vi "axis to can.vi"(4 "wej  ID":T4, 7 "output cluster 3":T1 {"zadany" format="%<%H:%M:%S\n%x>T"}, 10 "wej wagi":T3, 11 "wej ster":cluster{"Y axis":i32, "X axis":i32}) -> (0 "array of cans":T5[](array[typedef]) {"type" items=["CAN Data", "CAN Remote"]; "identifier" format="%.0x"}, 1 "current time":timestamp format="%<%I:%M:%S %p\n%x>T", 2 "pierwsz ramka":T5 {"type" items=["CAN Data", "CAN Remote"]; "identifier" format="%.0x"}, 3 "druga ramka":T5 {"type" items=["CAN Data", "CAN Remote"]; "identifier" format="%.0x"}, 5 "wyj pred":cluster{u16, u16, u16, u16, u16, u16} {"?" scale=0.0..65000.0; "?" scale=0.0..65000.0; "?" scale=0.0..65000.0; "?" scale=0.0..65000.0; "?" scale=0.0..65000.0; "?" scale=0.0..65000.0}, 6 "output cluster 2":T2, 9 "wyœlij":bool=TRUE)   [LabVIEW 2014]
uses:
  CANFrameControl.ctl
panel:
  in  "reset":bool
  out "x-y":dbl
  out "Time has Elapsed":bool
  out "Elapsed Time (s)":dbl
  out "zadany czas":bool
  out "AUTO ?":bool
  out "P 10":dbl(slide) scale=-66000.0..66000.0
  out "L 10":dbl(slide) scale=-66000.0..66000.0
  out "L 9":dbl(slide) scale=-66000.0..66000.0
  out "L 8":dbl(slide) scale=-66000.0..66000.0
  out "P 9":dbl(slide) scale=-66000.0..66000.0
  out "P 8":dbl(slide) scale=-66000.0..66000.0
  out "P 7":dbl(slide) scale=-66000.0..66000.0
  out "P 6":dbl(slide) scale=-66000.0..66000.0
  out "L 7":dbl(slide) scale=-66000.0..66000.0
  out "L 6":dbl(slide) scale=-66000.0..66000.0
  out "P 5":dbl(slide) scale=-66000.0..66000.0
  out "L 5":dbl(slide) scale=-66000.0..66000.0
  out "P 4":dbl
  out "L 4":dbl
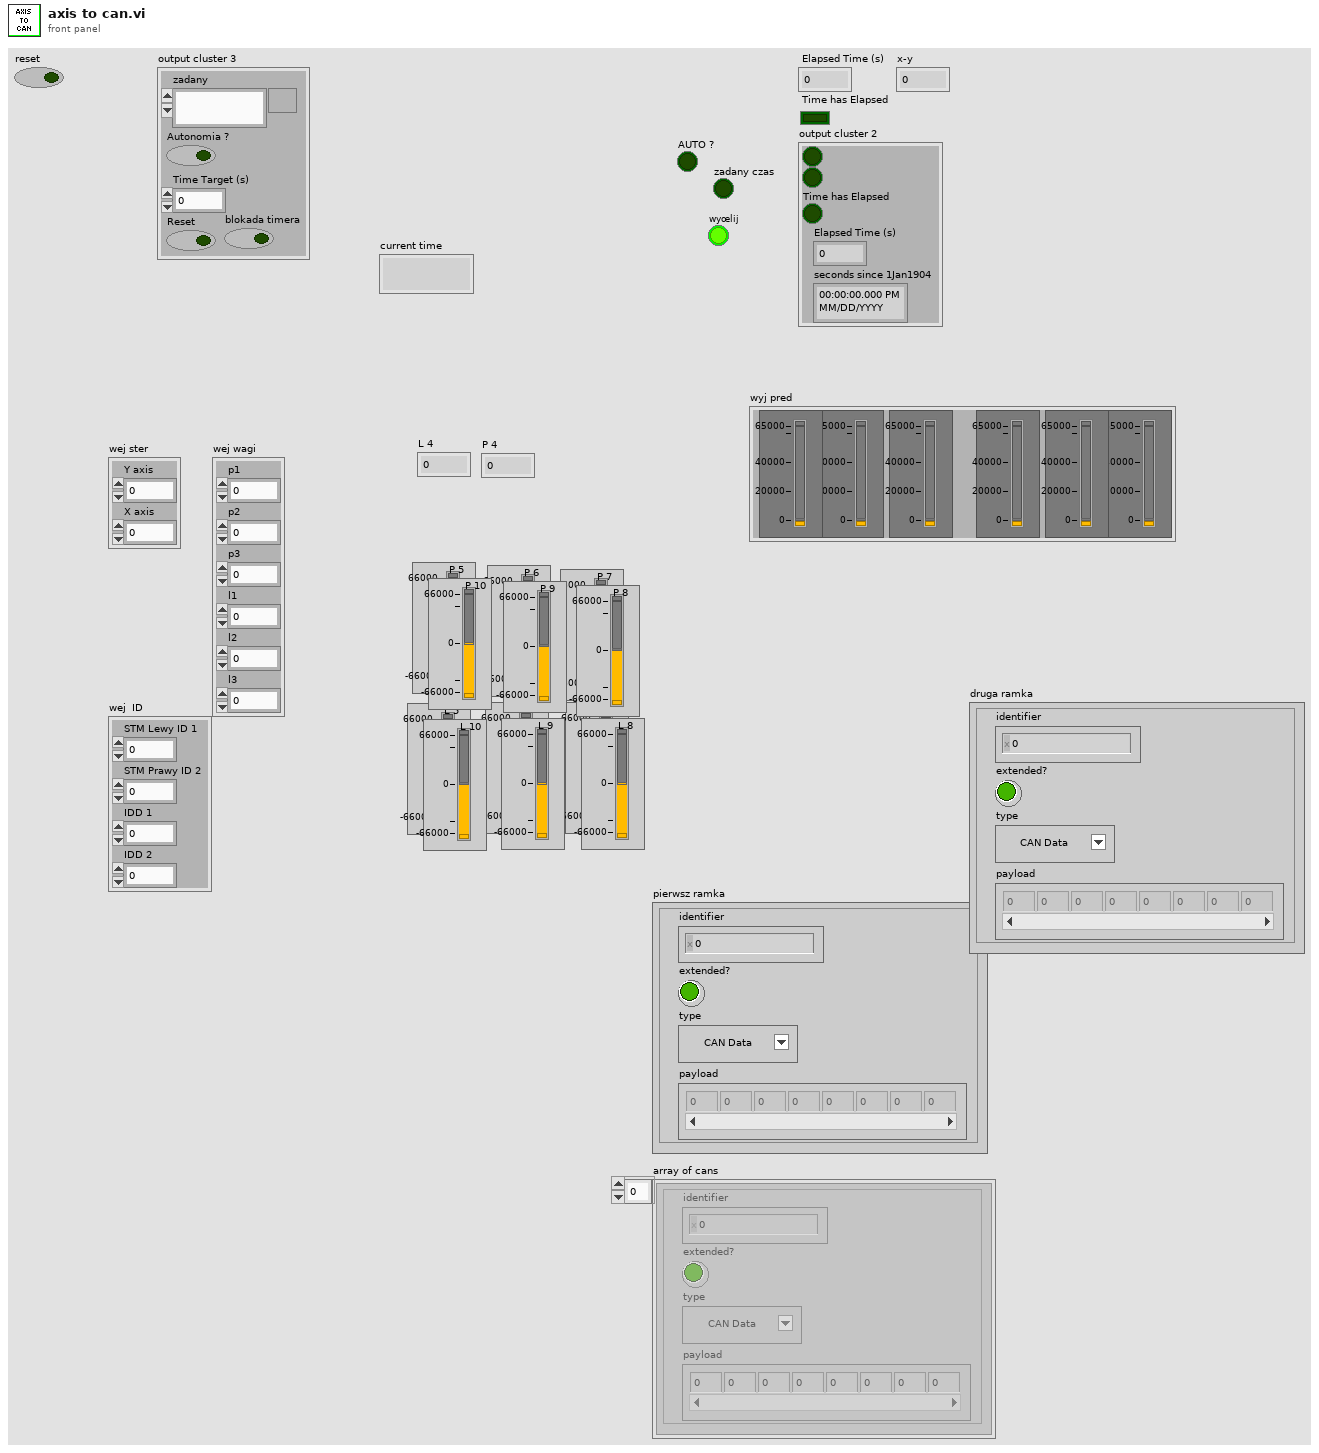
[diagram p1: front panel]
types:
  T1 = cluster{"zadany":timestamp, "Autonomia ?":bool, "Time Target (s)":dbl, "Reset":bool, "blokada timera":bool}
  T2 = cluster{bool, bool, "Time has Elapsed":bool, "Elapsed Time (s)":dbl, "seconds since 1Jan1904":timestamp}
  T3 = cluster{"p1":dbl, "p2":dbl, "p3":dbl, "l1":dbl, "l2":dbl, "l3":dbl}
  T4 = cluster{"STM Lewy ID 1":u32, "STM Prawy ID 2":u32, "IDD 1":u8, "IDD 2":u8}
  T5 = typedef "CANFrameControl.ctl" = cluster{"identifier":u32, "extended?":bool, "type":u8, "payload":u8[]}
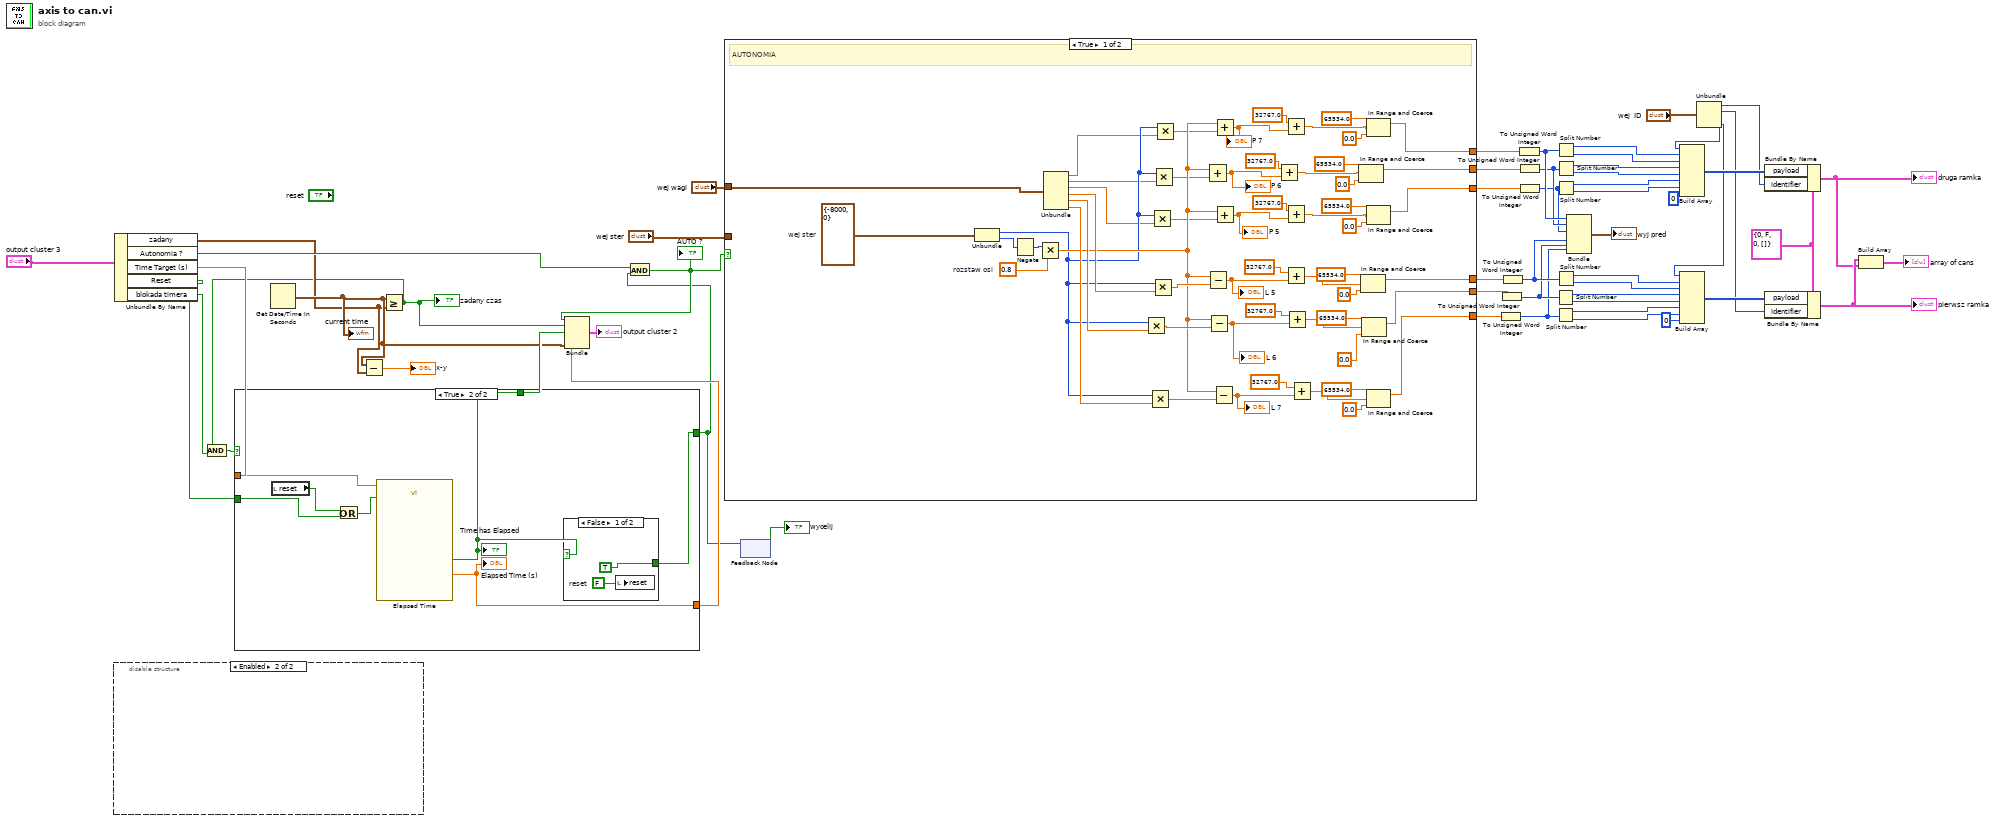
[diagram p0: block diagram]
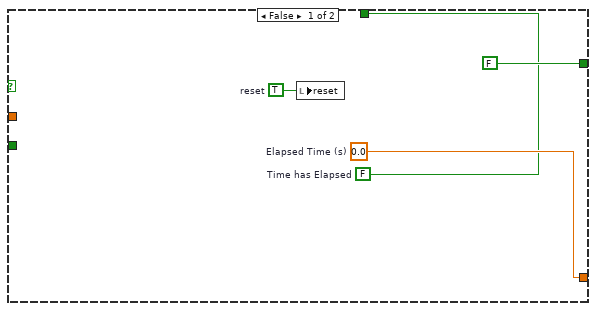
[diagram p2: hidden frame]
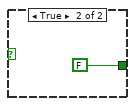
[diagram p3: hidden frame]
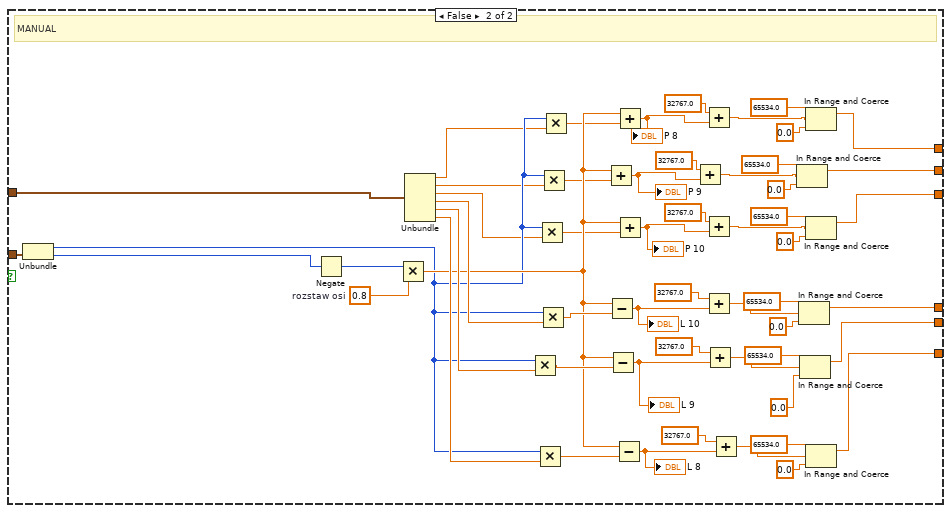
[diagram p4: hidden frame]
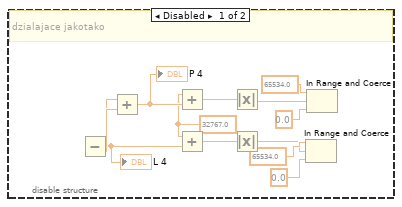
[diagram p5: hidden frame]
diagram:
  w55 = T5 {"identifier"=0, "extended?"=FALSE, "type"=0, "payload"=[]} ("CAN frame 2")
  n1 = disable-structure shown="Enabled" {
    frame Disabled {
      w59 = 32767.0 ("y")
      # "dzialajace jakotako"
      n2 = Add() -> (x=w69:dbl, y=w70:dbl, x+y=w66:dbl)
      "P 4" <- w66
      n3 = Subtract(x=w69, y=w70) -> (x-y=w67:dbl)
      "L 4" <- w67
      n4 = Add(x=w59, y=w66) -> (x+y=w58:dbl)
      n5 = Add(x=w59, y=w67) -> (x+y=w57:dbl)
      n6 = Absolute Value(x=w58) -> (abs(x)=w60:dbl)
      n7 = Absolute Value(x=w57) -> (abs(x)=w61:dbl)
      n8 = In Range and Coerce(upper limit=65534.0 ("y"), x=w61, lower limit=0.0 ("y")) -> ()  [unwired: 2 out]
      n9 = In Range and Coerce(upper limit=65534.0 ("y"), x=w60, lower limit=0.0 ("y")) -> (coerced(x)=w68:dbl)  [unwired: 1 out]
    }
    frame Enabled {
    }
  }
  n10 = Unbundle By Name("output cluster 3") -> ("zadany"=w8:timestamp, "Autonomia ?"=w12:bool, "Time Target (s)"=w11:dbl, "Reset"=w10:bool, "blokada timera"=w1:bool)
  n11 = Get Date/Time In Seconds() -> (seconds since 1Jan1904=w9:timestamp)
  "current time" <- w9
  n12 = Subtract(x=w9, y=w8) -> (x-y=→"x-y":dbl)
  n13 = Greater Or Equal?(x=w9, y=w8) -> (x >= y?=w3:bool)
  "zadany czas" <- w3
  n14 = And(x=w3, y=w1) -> (x .and. y?=w4:bool)
  n15 = case shown="True" w4 {
    tunnel: [FALSE w81] -> w5
    tunnel: [w72 w80] -> w15
    tunnel: [w73 w79] -> w14
    tunnel: w10 -> [_ w76]
    tunnel: w11 -> [_ w78]
    frame False {
      w71 = TRUE  # reset
      w73 = 0.0  # Elapsed Time (s)
      w72 = FALSE  # Time has Elapsed
      n16 = local write "reset"(w71) -> ()
    }
    frame True {
      n17 = local read "reset"() -> (w75:bool)
      n18 = Or(x=w75, y=w76) -> (x .or. y?=w77:bool)
      n19 = call "Elapsed Time"("Time Target (s)"=w78, "Reset"=w77) -> ("Elapsed Time (s)"=w79:dbl, "Time has Elapsed"=w80:bool)  [unwired: 10 in, 6 out]
      "Elapsed Time (s)" <- w79
      "Time has Elapsed" <- w80
      n20 = case shown="False" w80 {
        tunnel: [TRUE FALSE] -> w81
        frame False {
          w82 = FALSE  # reset
          n21 = local write "reset"(w82) -> ()
        }
        frame True {
        }
      }
    }
  }
  n22 = And(x=w12, y=w5) -> (x .and. y?=w16:bool)
  "AUTO ?" <- w16
  n23 = Bundle(w16, w3, "Time has Elapsed"=w15, "Elapsed Time (s)"=w14, "seconds since 1Jan1904"=w9) -> (→"output cluster 2":T2)  [unwired: 1 in]
  n24 = case shown="True" w16 {
    tunnel: [w113 w168] -> w24
    tunnel: [w112 w167] -> w23
    tunnel: [w111 w166] -> w22
    tunnel: [w97 w152] -> w21
    tunnel: [w96 w151] -> w20
    tunnel: [w95 w150] -> w19
    tunnel: "wej ster" -> [_ w141]
    tunnel: "wej wagi" -> [w86 w140]
    frame True {
      w85 = cluster{"Y axis":i32, "X axis":i32} {"Y axis"=-8000, "X axis"=0}  # wej ster
      w134 = 0.8  # rozstaw osi
      # "AUTONOMIA"
      n25 = Unbundle(w85) -> ("Y axis"=w93:i32, "X axis"=w133:i32)
      n26 = Negate(x=w133) -> (-x=w132:i32)
      n27 = Multiply(x=w132, y=w134) -> (x*y=w94:dbl)
      n28 = Unbundle(w86) -> ("p1"=w92:dbl, "p2"=w91:dbl, "p3"=w90:dbl, "l1"=w110:dbl, "l2"=w109:dbl, "l3"=w108:dbl)
      n29 = Multiply(x=w93, y=w109) -> (x*y=w115:dbl)
      n30 = Multiply(x=w93, y=w108) -> (x*y=w114:dbl)
      n31 = Multiply(x=w93, y=w90) -> (x*y=w87:dbl)
      n32 = Multiply(x=w93, y=w110) -> (x*y=w116:dbl)
      n33 = Multiply(x=w93, y=w91) -> (x*y=w88:dbl)
      n34 = Multiply(x=w93, y=w92) -> (x*y=w89:dbl)
      n35 = Add(x=w94, y=w88) -> (x+y=w106:dbl)
      "P 6" <- w106
      n36 = Subtract(x=w94, y=w116) -> (x-y=w130:dbl)
      "L 5" <- w130
      n37 = Subtract(x=w94, y=w115) -> (x-y=w124:dbl)
      "L 6" <- w124
      n38 = Subtract(x=w94, y=w114) -> (x-y=w119:dbl)
      "L 7" <- w119
      n39 = Add(x=w94, y=w89) -> (x+y=w99:dbl)
      "P 7" <- w99
      n40 = Add(x=w94, y=w87) -> (x+y=w131:dbl)
      "P 5" <- w131
      n41 = Add(x=32767.0 ("y"), y=w106) -> (x+y=w107:dbl)
      n42 = Add(x=32767.0 ("y"), y=w99) -> (x+y=w98:dbl)
      n43 = Add(x=32767.0 ("y"), y=w131) -> (x+y=w128:dbl)
      n44 = Add(x=32767.0 ("y"), y=w130) -> (x+y=w129:dbl)
      n45 = Add(x=32767.0 ("y"), y=w124) -> (x+y=w125:dbl)
      n46 = Add(x=32767.0 ("y"), y=w119) -> (x+y=w118:dbl)
      n47 = In Range and Coerce(upper limit=65534.0 ("y"), x=w107, lower limit=0.0 ("y")) -> (coerced(x)=w96:dbl)  [unwired: 1 out]
      n48 = In Range and Coerce(upper limit=65534.0 ("y"), x=w129, lower limit=0.0 ("y")) -> (coerced(x)=w113:dbl)  [unwired: 1 out]
      n49 = In Range and Coerce(upper limit=65534.0 ("y"), x=w125, lower limit=0.0 ("y")) -> (coerced(x)=w112:dbl)  [unwired: 1 out]
      n50 = In Range and Coerce(upper limit=65534.0 ("y"), x=w98, lower limit=0.0 ("y")) -> (coerced(x)=w95:dbl)  [unwired: 1 out]
      n51 = In Range and Coerce(upper limit=65534.0 ("y"), x=w128, lower limit=0.0 ("y")) -> (coerced(x)=w97:dbl)  [unwired: 1 out]
      n52 = In Range and Coerce(upper limit=65534.0 ("y"), x=w118, lower limit=0.0 ("y")) -> (coerced(x)=w111:dbl)  [unwired: 1 out]
    }
    frame False {
      w189 = 0.8  # rozstaw osi
      # "MANUAL"
      n53 = Unbundle(w141) -> ("Y axis"=w148:i32, "X axis"=w188:i32)
      n54 = Negate(x=w188) -> (-x=w187:i32)
      n55 = Multiply(x=w187, y=w189) -> (x*y=w149:dbl)
      n56 = Unbundle(w140) -> ("p1"=w147:dbl, "p2"=w146:dbl, "p3"=w145:dbl, "l1"=w165:dbl, "l2"=w164:dbl, "l3"=w163:dbl)
      n57 = Multiply(x=w148, y=w164) -> (x*y=w170:dbl)
      n58 = Multiply(x=w148, y=w163) -> (x*y=w169:dbl)
      n59 = Multiply(x=w148, y=w145) -> (x*y=w142:dbl)
      n60 = Multiply(x=w148, y=w165) -> (x*y=w171:dbl)
      n61 = Multiply(x=w148, y=w146) -> (x*y=w143:dbl)
      n62 = Multiply(x=w148, y=w147) -> (x*y=w144:dbl)
      n63 = Add(x=w149, y=w143) -> (x+y=w161:dbl)
      "P 9" <- w161
      n64 = Subtract(x=w149, y=w171) -> (x-y=w185:dbl)
      "L 10" <- w185
      n65 = Subtract(x=w149, y=w170) -> (x-y=w179:dbl)
      "L 9" <- w179
      n66 = Subtract(x=w149, y=w169) -> (x-y=w174:dbl)
      "L 8" <- w174
      n67 = Add(x=w149, y=w144) -> (x+y=w154:dbl)
      "P 8" <- w154
      n68 = Add(x=w149, y=w142) -> (x+y=w186:dbl)
      "P 10" <- w186
      n69 = Add(x=32767.0 ("y"), y=w161) -> (x+y=w162:dbl)
      n70 = Add(x=32767.0 ("y"), y=w154) -> (x+y=w153:dbl)
      n71 = Add(x=32767.0 ("y"), y=w186) -> (x+y=w183:dbl)
      n72 = Add(x=32767.0 ("y"), y=w185) -> (x+y=w184:dbl)
      n73 = Add(x=32767.0 ("y"), y=w179) -> (x+y=w180:dbl)
      n74 = Add(x=32767.0 ("y"), y=w174) -> (x+y=w173:dbl)
      n75 = In Range and Coerce(upper limit=65534.0 ("y"), x=w162, lower limit=0.0 ("y")) -> (coerced(x)=w151:dbl)  [unwired: 1 out]
      n76 = In Range and Coerce(upper limit=65534.0 ("y"), x=w184, lower limit=0.0 ("y")) -> (coerced(x)=w168:dbl)  [unwired: 1 out]
      n77 = In Range and Coerce(upper limit=65534.0 ("y"), x=w180, lower limit=0.0 ("y")) -> (coerced(x)=w167:dbl)  [unwired: 1 out]
      n78 = In Range and Coerce(upper limit=65534.0 ("y"), x=w153, lower limit=0.0 ("y")) -> (coerced(x)=w150:dbl)  [unwired: 1 out]
      n79 = In Range and Coerce(upper limit=65534.0 ("y"), x=w183, lower limit=0.0 ("y")) -> (coerced(x)=w152:dbl)  [unwired: 1 out]
      n80 = In Range and Coerce(upper limit=65534.0 ("y"), x=w173, lower limit=0.0 ("y")) -> (coerced(x)=w166:dbl)  [unwired: 1 out]
    }
  }
  n81 = feedback-in #1(w5) -> ()
  n82 = feedback #1() -> (→"wyœlij":bool)  [unwired: 1 in]
  n83 = To Unsigned Word Integer(number=w22) -> (unsigned 16bit integer=w26:u16)
  n84 = To Unsigned Word Integer(number=w23) -> (unsigned 16bit integer=w27:u16)
  n85 = To Unsigned Word Integer(number=w24) -> (unsigned 16bit integer=w28:u16)
  n86 = To Unsigned Word Integer(number=w19) -> (unsigned 16bit integer=w31:u16)
  n87 = To Unsigned Word Integer(number=w20) -> (unsigned 16bit integer=w30:u16)
  n88 = To Unsigned Word Integer(number=w21) -> (unsigned 16bit integer=w29:u16)
  n89 = Split Number(x=w27) -> (hi(x)=w40:u8, lo(x)=w39:u8)
  n90 = Split Number(x=w26) -> (hi(x)=w38:u8, lo(x)=w37:u8)
  n91 = Split Number(x=w31) -> (hi(x)=w50:u8, lo(x)=w49:u8)
  n92 = Split Number(x=w30) -> (hi(x)=w44:u8, lo(x)=w43:u8)
  n93 = Split Number(x=w29) -> (hi(x)=w42:u8, lo(x)=w41:u8)
  n94 = Split Number(x=w28) -> (hi(x)=w47:u8, lo(x)=w46:u8)
  n95 = Bundle(w31, w30, w29, w28, w27, w26) -> (→"wyj pred":cluster{u16, u16, u16, u16, u16, u16})  [unwired: 1 in]
  n96 = Unbundle("wej  ID") -> ("STM Lewy ID 1"=w35:u32, "STM Prawy ID 2"=w34:u32, "IDD 1"=w33:u8, "IDD 2"=w32:u8)
  n97 = Build Array(w33, w50, w49, w44, w43, w42, w41, u8 0 ("element")) -> (w54:u8[])
  n98 = Build Array(w32, w47, w46, w40, w39, w38, w37, u8 0 ("element")) -> (w56:u8[])
  n99 = Bundle By Name(cluster=w55, "payload"=w54, "identifier"=w35) -> (w52:T5)
  "druga ramka" <- w52
  n100 = Bundle By Name(cluster=w55, "payload"=w56, "identifier"=w34) -> (w53:T5)
  "pierwsz ramka" <- w53
  n101 = Build Array(w53, w52) -> (→"array of cans":T5[])
